vi "Get Sequence Return Value.vi"(8 "error in (no error)":errorcluster, 10 "Sequence Name":string, 11 "Session Ref in":T2) -> (0 "error out":errorcluster, 1 "Data Value Ref":T1, 2 "Sequence Name out":string, 3 "Session Ref out":T2)   [LabVIEW 2020, in "NI_VS Sequence Execution Interface.lvlib"]
doc: "Returns a reference to the return value of a sequence. The sequence must be complete or this VI returns an error."
uses:
  <vilib>/NI VeriStand/Execution/SequenceExecutionInterface/NI_VS Sequence Execution Interface.lvlib
  <vilib>/NI VeriStand/Execution/SequenceExecutionInterface/Stimulus Profile Session Ref.ctl
  NationalInstruments.VeriStand.ClientAPI
  <vilib>/NI VeriStand/Execution/SequenceExecutionInterface/Data Value Ref.ctl
  NationalInstruments.VeriStand.DataTypes
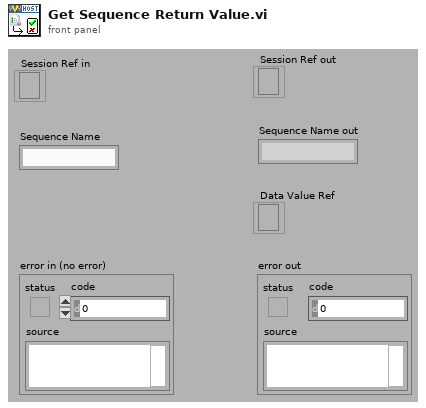
[diagram p1: front panel]
types:
  T1 = typedef "NI_VS Sequence Execution Interface.lvlib/Data Value Ref.ctl" = refnum<k24>
  T2 = typedef "NI_VS Sequence Execution Interface.lvlib/Stimulus Profile Session Ref.ctl" = refnum<k24>
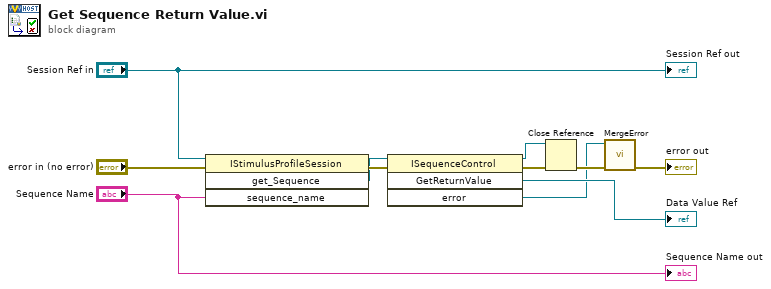
[diagram p0: block diagram]
diagram:
  n1 = invoke class="IStimulusProfileSession" method="get_Sequence"(reference="Session Ref in", error in="error in (no error)", "sequence_name"="Sequence Name") -> (error out=w8:errorcluster, "get_Sequence"=w6:refnum<k24>)  [unwired: 1 in, 2 out]
  n2 = invoke class="ISequenceControl" method="GetReturnValue"(reference=w6, error in=w8) -> (reference out=w5:refnum<k24>, error out=w7:errorcluster, "GetReturnValue"=→"Data Value Ref":refnum<k24>, "error"=w1:refnum<k24>)  [unwired: 2 in]
  n3 = Close Reference(reference=w5, error in (no error)=w7) -> (error out=w3:errorcluster)
  n4 = call <vilib>:"MergeError.vi"("error in (no error)"=w3, "Error"=w1) -> ("error out"=→"error out":errorcluster)  [unwired: 9 out]
  "Session Ref out" <- "Session Ref in"
  "Sequence Name out" <- "Sequence Name"
